vi "Run.vi"(8 "error in (no error)":errorcluster, 9 "Time Ratio used":dbl, 10 "Maze (0: Empty, -1: Enemy. >0: Teammate":i32[][](array[numeric]), 11 "Snail In":refnum<class "Random Location.lvclass">) -> (0 "error out":errorcluster, 1 "Direction":T1, 2 "Action":T2, 3 "Snail Out":refnum<class "Random Location.lvclass">, 4 "Replicated":refnum<class "Square.lvclass">)   [LabVIEW 2015, in "Random Location.lvclass"]
uses:
  Random Location.lvclass
  Type Defs/Action Enum.ctl
  Type Defs/Direction Enum.ctl
  Square/Square.lvclass
  Random Location.lvclass/Random Location.ctl
  Common/Reverse Direction.vi
  SubVIs/Read-Only Globals.vi
  Type Defs/SB Type Defs.lvlib
  Common/Common.lvlib
panel:
  # "NOTICE - YOU MUST NOT REMOVE THIS NOTICE. PER THE FOLLOWING LICENSE, YOU MAY REPRODUCE THIS SOFTWARE PROVIDED YOU FOLLOW THE TERMS\nOF THE LICENSE.\n\n---BEGIN BSD LICENSE (http://opensource.org/licenses/BSD-2-Clause)---\nCopyright (c) 2015, Endigit, Inc. <robert@endigit.com>\nAll rights reserved.\n\nRedistribution and use in source and binary forms, with or without modification, are permitted provided that the following conditions are met:\n\n1. Redistributions of source code must retain the above copyright notice, this list of conditions and the following disclaimer.\n\n2. Redistributions in binary form must reproduce the above copyright notice, this list of conditions and the following disclaimer in the documentation and/or other \nmaterials provided with the distribution.\n\nTHIS SOFTWARE IS PROVIDED BY THE COPYRIGHT HOLDERS AND CONTRIBUTORS \"AS IS\" AND ANY EXPRESS OR IMPLIED WARRANTIES, INCLUDING, BUT NOT \nLIMITED TO, THE IMPLIED WARRANTIES OF MERCHANTABILITY AND FITNESS FOR A PARTICULAR PURPOSE ARE DISCLAIMED. IN NO EVENT SHALL THE COPYRIGHT \nHOLDER OR CONTRIBUTORS BE LIABLE FOR ANY DIRECT, INDIRECT, INCIDENTAL, SPECIAL, EXEMPLARY, OR CONSEQUENTIAL DAMAGES (INCLUDING, BUT NOT \nLIMITED TO, PROCUREMENT OF SUBSTITUTE GOODS OR SERVICES; LOSS OF USE, DATA, OR PROFITS; OR BUSINESS INTERRUPTION) HOWEVER CAUSED AND ON \nANY THEORY OF LIABILITY, WHETHER IN CONTRACT, STRICT LIABILITY, OR TORT (INCLUDING NEGLIGENCE OR OTHERWISE) ARISING IN ANY WAY OUT OF THE USE \nOF THIS SOFTWARE, EVEN IF ADVISED OF THE POSSIBILITY OF SUCH DAMAGE.\n---END BSD LICENSE---"
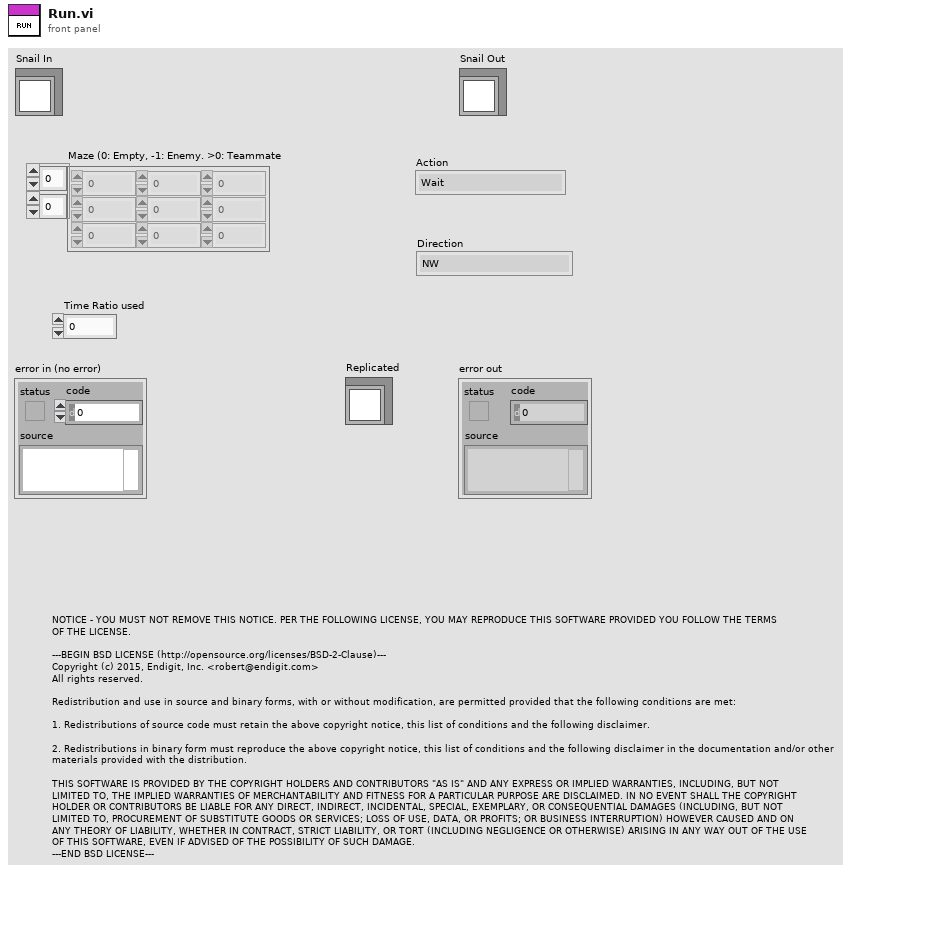
[diagram p1: front panel]
types:
  T1 = typedef "SB Type Defs.lvlib/Direction Enum.ctl" = enum16{"NW", "N", "NE", "E", "SE", "S", "SW", "W"}
  T2 = typedef "SB Type Defs.lvlib/Action Enum.ctl" = enum16{"Wait", "Move", "Attack", "Replicate"}
  T3 = typedef "Common.lvlib/Position.ctl" = cluster{"Column":i32, "Row":i32}
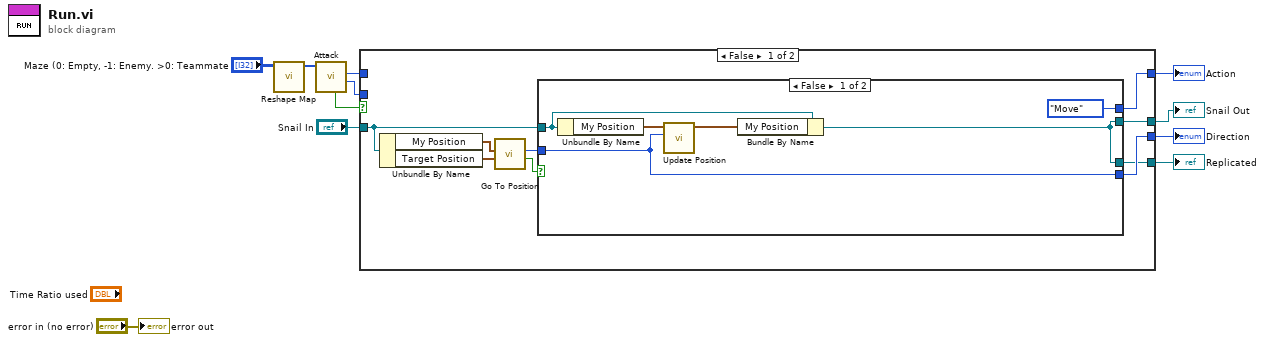
[diagram p0: block diagram]
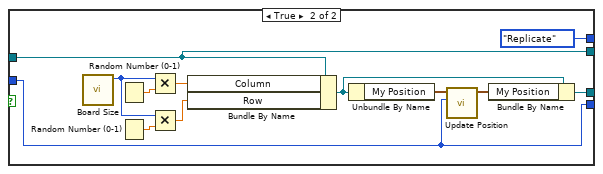
[diagram p2: hidden frame]
diagram:
  n1 = call "Reshape Map.vi"("Maze (0: Empty, -1: Enemy. >0: Teammate"="Maze (0: Empty, -1: Enemy. >0: Teammate") -> ("Map"=w6:i32[])  [unwired: 9 in, 1 out]
  n2 = call "Attack.vi"("Maze (0: Empty, -1: Enemy. >0: Teammate"=w6) -> ("Direction"=w2:i32, "Action"=w3:T2, "Enemy Found?"=w4:bool)  [unwired: 5 in, 3 out]
  n3 = case shown="False" w4 {
    tunnel: [w18 w41] -> w9
    tunnel: "Snail In" -> [w17 w39]
    tunnel: [w12 w39] -> w7
    tunnel: [w14 w40] -> w5
    tunnel: w3 -> [_ w41]
    tunnel: w2 -> [_ w40]
    tunnel: [w13 w39] -> w1
    frame False {
      n4 = Unbundle By Name(w17) -> ("My Position"=w20:cluster{"Column":i32, "Row":i32}, "Target Position"=w19:cluster{"Column":i32, "Row":i32})
      n5 = call "Go To Position.vi"("Target Position"=w19, "My Position"=w20) -> ("Arrived?"=w16:bool, "Direction"=w15:T1)  [unwired: 7 in, 1 out]
      n6 = case shown="False" w16 {
        tunnel: [Action_Enum."Move" ("f") Action_Enum."Replicate" ("x")] -> w18
        tunnel: w17 -> [w24 w27]
        tunnel: [w21 w27] -> w13
        tunnel: w15 -> [w22 w29]
        tunnel: [w22 w29] -> w14
        tunnel: [w21 w28] -> w12
        frame False {
          n7 = Unbundle By Name(w24) -> ("My Position"=w25:cluster{"Column":i32, "Row":i32})
          n8 = call "Update Position.vi"("Direction"=w22, "Position in"=w25) -> ("Position out"=w23:T3)  [unwired: 9 in]
          n9 = Bundle By Name(cluster=w24, "My Position"=w23) -> (w21:refnum<class "Random Location.lvclass">)
        }
        frame True {
          n10 = call "Board Size.vi"() -> ("Board Size"=w36:i32)  [unwired: 11 in]
          n11 = Random Number (0-1)() -> (number: 0 to 1=w35:dbl)
          n12 = Random Number (0-1)() -> (number: 0 to 1=w37:dbl)
          n13 = Multiply(x=w36, y=w35) -> (x*y=w34:dbl)
          n14 = Multiply(x=w36, y=w37) -> (x*y=w33:dbl)
          n15 = Bundle By Name(cluster=w27, "Column"=w34, "Row"=w33) -> (w32:refnum<class "Random Location.lvclass">)
          n16 = Unbundle By Name(w32) -> ("My Position"=w31:cluster{"Column":i32, "Row":i32})
          n17 = call "Update Position.vi"("Direction"=w29, "Position in"=w31) -> ("Position out"=w30:T3)  [unwired: 9 in]
          n18 = Bundle By Name(cluster=w32, "My Position"=w30) -> (w28:refnum<class "Random Location.lvclass">)
        }
      }
    }
    frame True {
    }
  }
  "Snail Out" <- w1
  "Action" <- w9
  "Replicated" <- w7
  "Direction" <- w5
  "error out" <- "error in (no error)"
